vi "nearest multiple.vi"(9 "y":dbl, 10 "x":dbl) -> (1 "INT32(round(x/y)*y)":i32, 2 "round(x/y)*y":dbl, 4 "index":i32)   [LabVIEW 2020]
panel:
  # "Computes nearest multiple"
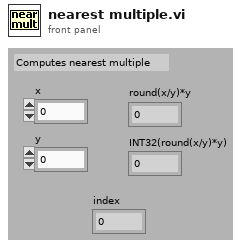
[diagram p1: front panel]
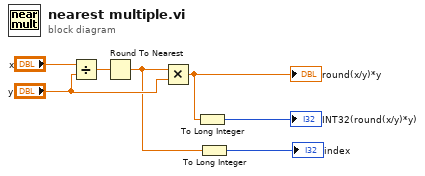
[diagram p0: block diagram]
diagram:
  n1 = Divide(x="x", y="y") -> (x/y=w7:dbl)
  n2 = Round To Nearest(number=w7) -> (nearest integer value=w1:dbl)
  n3 = Multiply(x=w1, y="y") -> (x*y=w3:dbl)
  "round(x/y)*y" <- w3
  n4 = To Long Integer(number=w3) -> (32bit integer=→"INT32(round(x/y)*y)":i32)
  n5 = To Long Integer(number=w1) -> (32bit integer=→"index":i32)
